vi "DependencyInspector.vi"() -> ()   [LabVIEW 2020]
uses:
  DependencyInspection/CItemMatch/TypeDefs/Field.ctl
  DependencyInspection/CItemMatch/TypeDefs/ComparisonType.ctl
  ExtensionInterfaces/IConfigurationPage/Event_ParametersRef.ctl
  ExtensionInterfaces/IConfigurationPage/Event_Parameters.ctl
  DependencyInspection/CDependencyInspector/CDependencyInspection.lvclass
  UIManager/UIManager.lvclass
  DependencyInspection/CDependencyInspector/Options.ctl
  DependencyInspection/CDependencyInspector/Options_Export.ctl
  DependencyInspection/CDependencyInspector/Options_Filter.ctl
  DependencyInspection/CItemMatch/CItemMatch.lvclass
  ExtensionInterfaces/IConfigurationPage/IConfigurationPage.lvclass
  DependencyInspector.lvlib
panel:
  in  "Tab Control":T1(tab)
  in  "Target filter":T4
  in  "Source filter":T4
  in  "Circular deps":bool
  in  "Top level only":bool
  in  "Tests into a separate group":bool
  in  "Path to Check":path
  in  "Exclude instances":bool=TRUE
  in  "Exclude external":bool=TRUE
  in  "Root Path":path
  in  "AND Condition?":bool
  in  "Rules parsers":string(combo)
  in  "Export Rules":bool=TRUE
  in  "Export Dependencies":bool=TRUE
  in  "Exporters":string(combo)
  in  "Export Invalid Dependencies":bool=TRUE
  in  "Export Concessions":bool=TRUE
  in  "Export Undeclared":bool=TRUE
  out "Results":string[][](table)
  out "Number of Files":i32=286
  out "Linker Time (m)":dbl=0.015333333333333332 format="%#_6f"
  out "XML Time (m)":dbl format="%#_6f"
  out "File Time (m)":dbl format="%#_6f"
  in  "Close":bool
  in  "Run":bool
  # "Options"
  # "Options"
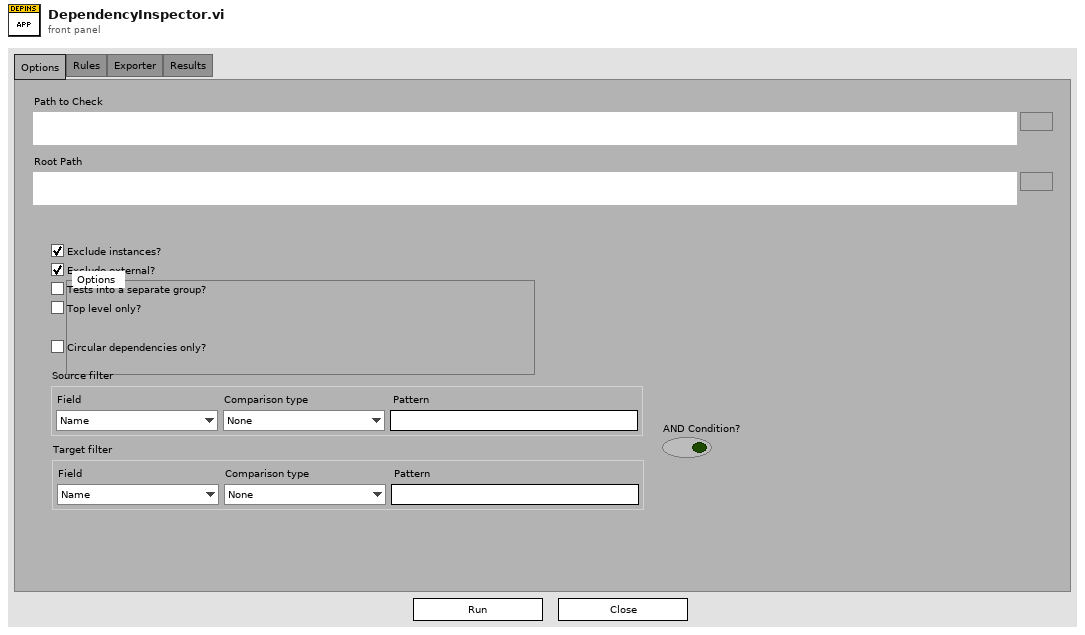
[diagram p1: front panel]
types:
  T1 = enum32{"Options", "Rules", "Exporter", "Results"}
  T2 = typedef "DependencyInspection.lvlib/CItemMatch.lvclass/Field.ctl" = enum16{"Name", "Qualified name", "Path"}
  T3 = typedef "DependencyInspection.lvlib/CItemMatch.lvclass/ComparisonType.ctl" = enum16{"None", "Ends with", "Equals", "Not equal", "Starts with", "Contains", "Matches pattern"}
  T4 = cluster{"Field":T2, "Comparison type":T3, "Pattern":string}
  T5 = typedef "ExtensionInterfaces.lvlib/IConfigurationPage.lvclass/Event_ParametersRef.ctl" = refnum<user-event>
  T6 = typedef "DependencyInspection.lvlib/CDependencyInspection.lvclass/Options.ctl" = cluster{"exclude instances?":bool, "exclude external? (T)":bool, "separate tests?":bool, "top level results only?":bool, "Export options":T7, "Filter options":T8}
  T7 = typedef "DependencyInspection.lvlib/CDependencyInspection.lvclass/Options_Export.ctl" = cluster{"Export rules":bool, "Export dependencies":bool, "Export invalid dependencies":bool, "Export concessions":bool, "Export undeclared":bool}
  T8 = typedef "DependencyInspection.lvlib/CDependencyInspection.lvclass/Options_Filter.ctl" = cluster{"Source filter":refnum<class "CItemMatch.lvclass">, "Target filter":refnum<class "CItemMatch.lvclass">, "AND Condition?":bool}
  T9 = typedef "DependencyInspector.lvlib/subReferenceData.ctl" = cluster{"VI Ref":refnum<vi>, "Stop":refnum<user-event>, "Parameters":refnum<user-event>}
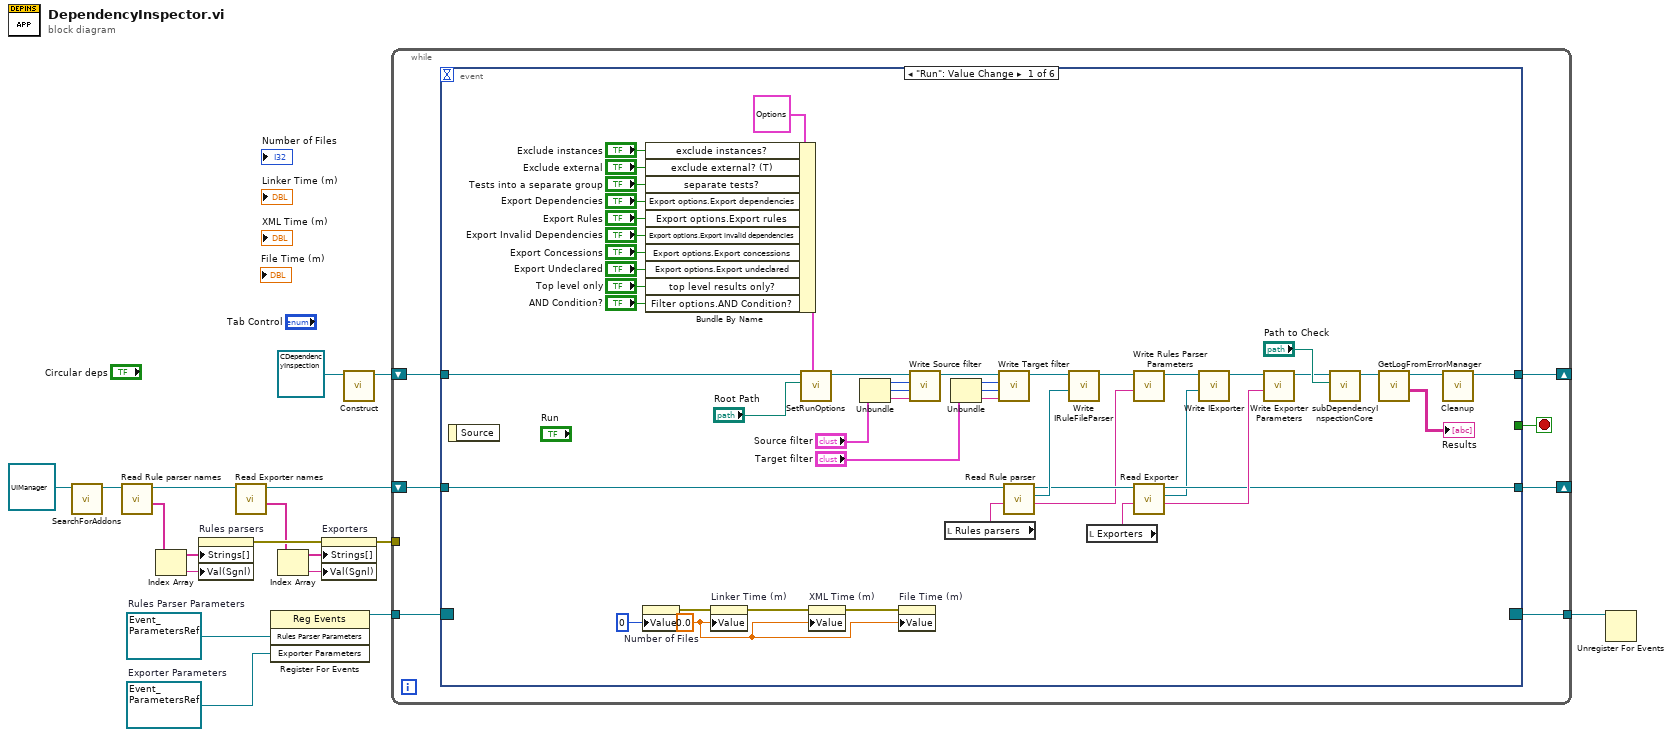
[diagram p0: block diagram]
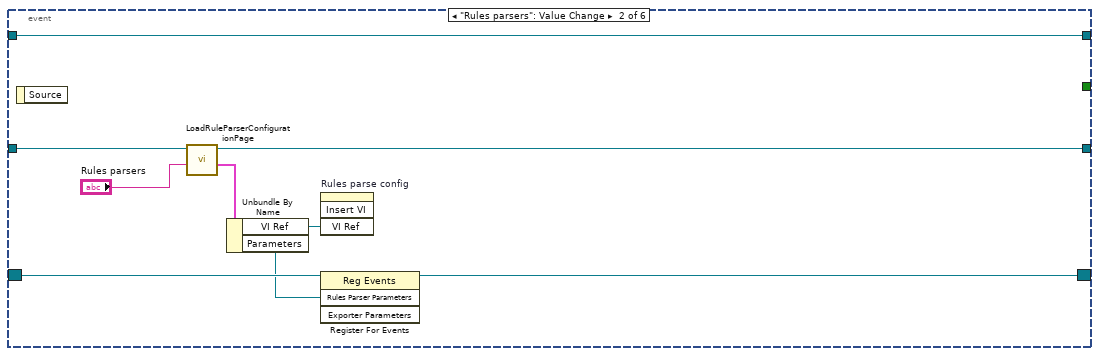
[diagram p2: hidden frame]
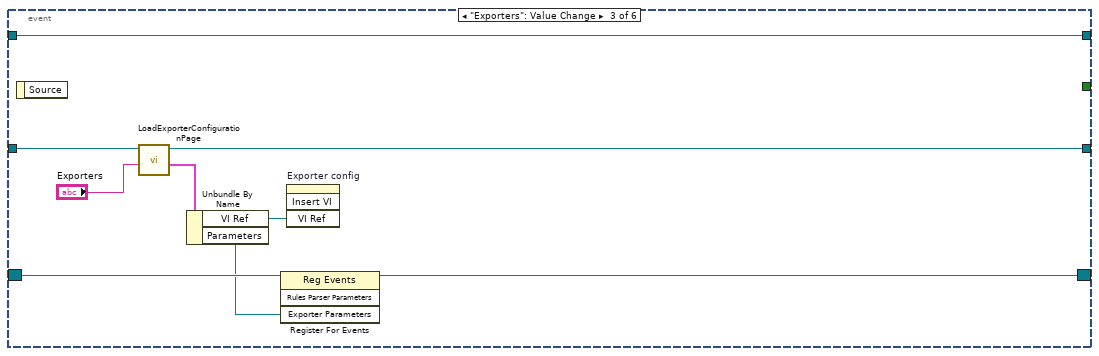
[diagram p3: hidden frame]
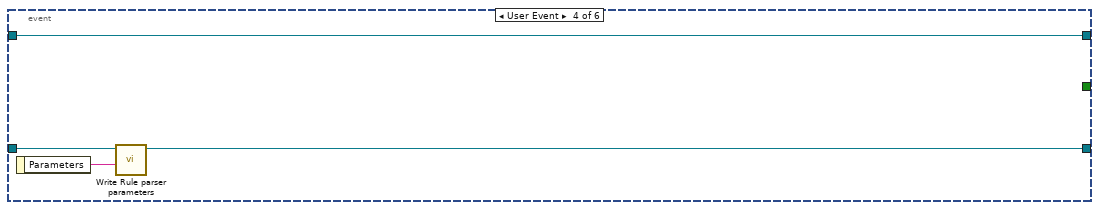
[diagram p4: hidden frame]
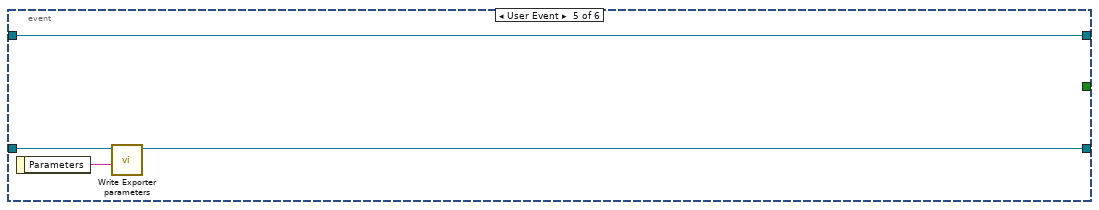
[diagram p5: hidden frame]
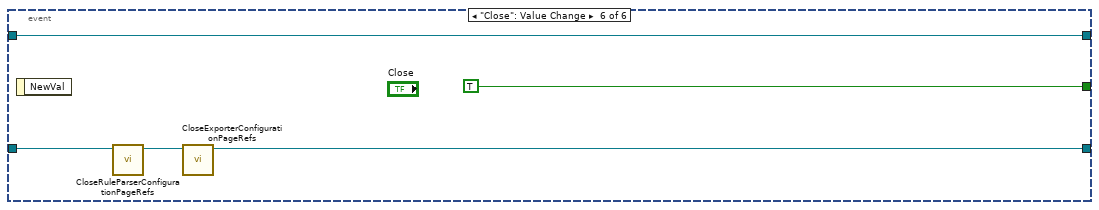
[diagram p6: hidden frame]
diagram:
  w11 = T5 refnum  # Exporter Parameters
  w15 = T5 refnum  # Rules Parser Parameters
  n1 = call-dynamic "SearchForAddons.vi"("UIManager in"=refnum<class "UIManager.lvclass"> refnum ("DependencyInspector.lvlib:UIManager.lvclass")) -> ("UIManager out"=w9:refnum<class "UIManager.lvclass">)  [unwired: 9 in, 1 out]
  n2 = call-dynamic "Read Rule parser names.vi"("UIManager in"=w9) -> ("Rule parser names"=w4:string[], "UIManager out"=w8:refnum<class "UIManager.lvclass">)  [unwired: 9 in]
  n3 = Index Array(array=w4) -> (element=w3:string)  [unwired: 1 in]
  n4 = property on="Rules parsers" class="CmbBox"("Strings[]"=w4, "Val(Sgnl)"=w3) -> (error out=w7:errorcluster)  [unwired: 2 in, 1 out]
  n5 = call-dynamic "Read Exporter names.vi"("UIManager in"=w8) -> ("Exporter names"=w2:string[], "UIManager out"=w5:refnum<class "UIManager.lvclass">)  [unwired: 9 in]
  n6 = register-events(w15, w11) -> (reference out=w16:refnum<event-registration>)  [unwired: 2 in, 1 out]
  n7 = Index Array(array=w2) -> (element=w1:string)  [unwired: 1 in]
  n8 = property on="Exporters" class="CmbBox"(error in=w7, "Strings[]"=w2, "Val(Sgnl)"=w1) -> (error out=w6:errorcluster)  [unwired: 1 in, 1 out]
  n9 = call-dynamic "Construct.vi"("CDependencyInspector in"=refnum<class "CDependencyInspection.lvclass"> refnum ("DGML_Generator_Helper.lvlib:CDependencyList.lvclass")) -> ("CDependencyInspector out"=w13:refnum<class "CDependencyInspection.lvclass">)  [unwired: 9 in, 1 out]
  n10 = while {
    tunnel: w16 -> [w22]
    shift-right: [w20] -> _
    shift-left: w13 -> [w21]
    tunnel: [w19] -> w12
    tunnel: w6 -> [_]
    shift-right: [w17] -> _
    shift-left: w5 -> [w18]
    stop <- w23 stop-if-true
    n11 = event shown="[0] \"Run\": Value Change" {
      selector: w22 -> [_ w80 w89 _ _ _]
      dyn-events: [_ w79 w88 _ _ _] -> w19
      timeout: _ -> [_ _ _ _ _ _]
      tunnel: [_ _ _ _ _ TRUE] -> w23
      tunnel: w21 -> [w62 w76 w85 w90 w94 w101]
      tunnel: [w36 w76 w85 w90 w94 w101] -> w20
      tunnel: w18 -> [w52 w75 w83 w92 w96 w98]
      tunnel: [w43 w74 w84 w93 w97 w99] -> w17
      event "Run": Value Change {
        w65 = 0.0 ("Linker Time (m)")
        n12 = event-data() -> ()  [unwired: 1 in, 1 out]
        n13 = property on="Number of Files" class="DigNum (strict)"("Value"=0 ("Number of Files")) -> (error out=w68:errorcluster)  [unwired: 2 in, 1 out]
        n14 = Bundle By Name(cluster=T6 {"exclude instances?"=FALSE, "exclude external? (T)"=TRUE, "separate tests?"=FALSE, "top level results only?"=FALSE, "Export options"={"Export rules"=FALSE, "Export dependencies"=FALSE, "Export invalid dependencies"=FALSE, "Export concessions"=FALSE, "Export undeclared"=FALSE}, "Filter options"={"Source filter"=refnum, "Target filter"=refnum, "AND Condition?"=FALSE}} ("Options"), "exclude instances?"="Exclude instances", "exclude external? (T)"="Exclude external", "separate tests?"="Tests into a separate group", "Export options.Export dependencies"="Export Dependencies", "Export options.Export rules"="Export Rules", "Export options.Export invalid dependencies"="Export Invalid Dependencies", "Export options.Export concessions"="Export Concessions", "Export options.Export undeclared"="Export Undeclared", "top level results only?"="Top level only", "Filter options.AND Condition?"="AND Condition?") -> (w59:T6)
        n15 = property on="Linker Time (m)" class="DigNum (strict)"(error in=w68, "Value"=w65) -> (error out=w67:errorcluster)  [unwired: 1 in, 1 out]
        n16 = call-dynamic "SetRunOptions.vi"("Options"=w59, "Root path"="Root Path", "CDependencyInspection in"=w62) -> ("CDependencyInspection out"=w25:refnum<class "CDependencyInspection.lvclass">)  [unwired: 7 in, 1 out]
        n17 = property on="XML Time (m)" class="DigNum (strict)"(error in=w67, "Value"=w65) -> (error out=w66:errorcluster)  [unwired: 1 in, 1 out]
        n18 = Unbundle("Source filter") -> ("Field"=w32:T2, "Comparison type"=w31:T3, "Pattern"=w30:string)
        n19 = property on="File Time (m)" class="DigNum (strict)"(error in=w66, "Value"=w65) -> ()  [unwired: 1 in, 2 out]
        n20 = call-dynamic "Write Source filter.vi"("Filter"=w30, "Comparison type"=w31, "Field"=w32, "CDependencyInspection in"=w25) -> ("CDependencyInspection out"=w34:refnum<class "CDependencyInspection.lvclass">)  [unwired: 7 in]
        n21 = local read "Rules parsers"() -> (w41:string)
        n22 = Unbundle("Target filter") -> ("Field"=w28:T2, "Comparison type"=w27:T3, "Pattern"=w26:string)
        n23 = call-dynamic "Write Target filter.vi"("Filter"=w26, "Comparison type"=w27, "Field"=w28, "CDependencyInspection in"=w34) -> ("CDependencyInspection out"=w24:refnum<class "CDependencyInspection.lvclass">)  [unwired: 7 in]
        n24 = call-dynamic "Read Rule parser.vi"("Selection"=w41, "UIManager in"=w52) -> ("Parameters"=w45:string, "IRuleFileParser.lvclass"=w47:refnum<class "IRuleFileParser.lvclass">, "UIManager out"=w46:refnum<class "UIManager.lvclass">)  [unwired: 6 in, 1 out]
        n25 = call-dynamic "Write IRuleFileParser.vi"("IRuleFileParser"=w47, "CDependencyInspection in"=w24) -> ("CDependencyInspection out"=w51:refnum<class "CDependencyInspection.lvclass">)  [unwired: 9 in]
        n26 = local read "Exporters"() -> (w40:string)
        n27 = call-dynamic "Write Rules Parser Parameters.vi"("Parameters"=w45, "CDependencyInspection in"=w51) -> ("CDependencyInspection out"=w50:refnum<class "CDependencyInspection.lvclass">)  [unwired: 9 in]
        n28 = call-dynamic "Read Exporter.vi"("Selection"=w40, "UIManager in"=w46) -> ("Parameters"=w44:string, "IExporter.lvclass"=w42:refnum<class "IExporter.lvclass">, "UIManager out"=w43:refnum<class "UIManager.lvclass">)  [unwired: 6 in, 1 out]
        n29 = call-dynamic "Write IExporter.vi"("IExporter"=w42, "CDependencyInspection in"=w50) -> ("CDependencyInspection out"=w49:refnum<class "CDependencyInspection.lvclass">)  [unwired: 9 in]
        n30 = call-dynamic "Write Exporter Parameters.vi"("Parameters"=w44, "CDependencyInspection in"=w49) -> ("CDependencyInspection out"=w48:refnum<class "CDependencyInspection.lvclass">)  [unwired: 9 in]
        n31 = call "subDependencyInspectionCore.vi"("Path to Check"="Path to Check", "CDependencyInspection in"=w48) -> ("CDependencyInspection out"=w60:refnum<class "CDependencyInspection.lvclass">)  [unwired: 9 in]
        n32 = call-dynamic "GetLogFromErrorManager.vi"("CDependencyInspection in"=w60) -> ("Log results"=→"Results":string[][], "CDependencyInspection out"=w37:refnum<class "CDependencyInspection.lvclass">)  [unwired: 8 in, 1 out]
        n33 = call-dynamic "Cleanup.vi"("CDependencyInspection in"=w37) -> ("CDependencyInspection out"=w36:refnum<class "CDependencyInspection.lvclass">)  [unwired: 9 in, 1 out]
      }
      event "Rules parsers": Value Change {
        n34 = event-data() -> ()  [unwired: 1 in, 1 out]
        n35 = call-dynamic "LoadRuleParserConfigurationPage.vi"("Selection"="Rules parsers", "UIManager in"=w75) -> ("References"=w72:T9, "UIManager out"=w74:refnum<class "UIManager.lvclass">)  [unwired: 7 in, 1 out]
        n36 = Unbundle By Name(w72) -> ("VI Ref"=w78:refnum<vi>, "Parameters"=w77:refnum<user-event>)
        n37 = invoke on="Rules parse config" class="SubPnl" method="Insert VI"("VI Ref"=w78) -> ()  [unwired: 3 in, 4 out]
        n38 = register-events(reference=w80, w77) -> (reference out=w79:refnum<event-registration>)  [unwired: 2 in, 1 out]
      }
      event "Exporters": Value Change {
        n39 = event-data() -> ()  [unwired: 1 in, 1 out]
        n40 = call-dynamic "LoadExporterConfigurationPage.vi"("Selection"="Exporters", "UIManager in"=w83) -> ("References"=w81:T9, "UIManager out"=w84:refnum<class "UIManager.lvclass">)  [unwired: 7 in, 1 out]
        n41 = Unbundle By Name(w81) -> ("VI Ref"=w87:refnum<vi>, "Parameters"=w86:refnum<user-event>)
        n42 = register-events(reference=w89, w86) -> (reference out=w88:refnum<event-registration>)  [unwired: 2 in, 1 out]
        n43 = invoke on="Exporter config" class="SubPnl" method="Insert VI"("VI Ref"=w87) -> ()  [unwired: 3 in, 4 out]
      }
      event User Event {
        n44 = event-data() -> ("Parameters"=w91:string)  [unwired: 1 in]
        n45 = call-dynamic "Write Rule parser parameters.vi"("Parameters"=w91, "UIManager in"=w92) -> ("UIManager out"=w93:refnum<class "UIManager.lvclass">)  [unwired: 9 in]
      }
      event User Event {
        n46 = event-data() -> ("Parameters"=w95:string)  [unwired: 1 in]
        n47 = call-dynamic "Write Exporter parameters.vi"("Parameters"=w95, "UIManager in"=w96) -> ("UIManager out"=w97:refnum<class "UIManager.lvclass">)  [unwired: 9 in]
      }
      event "Close": Value Change {
        n48 = event-data() -> ()  [unwired: 1 in, 1 out]
        n49 = call "CloseRuleParserConfigurationPageRefs.vi"("UIManager in"=w98) -> ("UIManager out"=w100:refnum<class "UIManager.lvclass">)  [unwired: 9 in, 1 out]
        n50 = call "CloseExporterConfigurationPageRefs.vi"("UIManager in"=w100) -> ("UIManager out"=w99:refnum<class "UIManager.lvclass">)  [unwired: 9 in, 1 out]
      }
    }
  }
  n51 = Unregister For Events(event registration refnum=w12) -> ()  [unwired: 1 in, 1 out]
